vi "VS-Read All (standalone).vi"() -> (0 "error out":errorcluster, 1 "Heart Rate (bpm)":dbl, 2 "Temperature (C)":dbl)   [LabVIEW 2020]
uses:
  <vilib>/Utility/sysdir.llb/System Directory Type.ctl
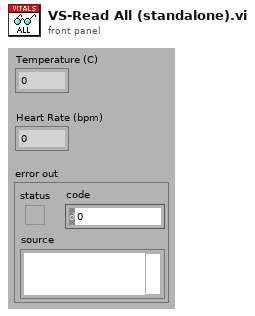
[diagram p1: front panel]
types:
  T1 = typedef "System Directory Type.ctl" = i32
  T2 = typedef "PhysMon-Options.ctl" = cluster{"Min Interval":dbl, "HR from ABR?":bool, "HR Scale":T3, "Temp Scale":T3, "Lock?":bool, "Temp Sensor":T4, "EKG":T5}
  T3 = typedef "PhysMon-Scale.ctl" = cluster{"Slope":dbl, "Offset":dbl, "Limits":cluster{"Min":dbl, "Max":dbl}, "term config":i32}
  T4 = typedef "PhysMon-TempSensor.ctl" = enum16{"YSI", "FHC", "Custom"}
  T5 = typedef "PhysMon-HR From EKG Settings.ctl" = cluster{"Sample duration (s)":dbl}
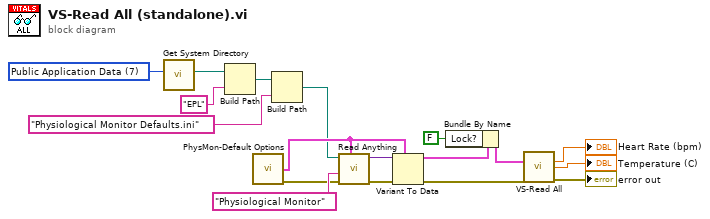
[diagram p0: block diagram]
diagram:
  w6 = T1 7 items=["User Home", "User Desktop", "User Documents", "User Application Data", "User Preferences", "User Temporary", "Public Documents", "Public Application Data", "Public Preferences", "System Core Libraries", "System Installed Libraries", "Application Files", "Boot Volume Root"] ("system directory type")
  n1 = call <vilib>:"Get System Directory.vi"("system directory type"=w6) -> ("system directory"=w5:path)  [unwired: 10 in]
  n2 = Build Path(base path=w5, name or relative path="EPL") -> (appended path=w3:path)
  n3 = call "PhysMon-Default Options.vi"() -> ("Options"=w13:T2, "error out"=w9:errorcluster)  [unwired: 14 in]
  n4 = Build Path(base path=w3, name or relative path="Physiological Monitor Defaults.ini") -> (appended path=w1:path)
  n5 = call "Read Anything.vi"("Type of Anything"=w13, "Error In"=w9, "Section Name (Name of \"Type of Anything\")"="Physiological Monitor" ("Section Name (Name of \"Type of Anything\")"), "Path (dialog)"=w1) -> ("Error Out"=w10:errorcluster, "Anything"=w12:variant)  [unwired: 5 in, 1 out]
  n6 = Variant To Data(error in=w10, type=w13, Variant=w12) -> (data=w14:T2, error out=w15:errorcluster)
  n7 = Bundle By Name(cluster=w14, "Lock?"=FALSE) -> (w8:T2)
  n8 = call "VS-Read All.vi"("Options"=w8, "error in (no error)"=w15) -> ("Heart Rate (bpm)"=→"Heart Rate (bpm)":dbl, "Temperature (C)"=→"Temperature (C)":dbl, "error out"=→"error out":errorcluster)  [unwired: 10 in, 1 out]
